vi "array -- bilinear regression 2D -- V1.vi"(7 "action":T2, 10 "fit  IN":dbl[](array[numeric])=[1.9, 2.6, 3.3, 1.0, 2.7, 3.9], 11 "xyz IN":cluster{"x":dbl[], "y":dbl[], "z":dbl[]}={"x"=[0.0, 0.0, 0.0, -1.0, -1.0, -1.0, 1.0, 1.0, 1.0], "y"=[-1.0, 0.0, 1.0, -1.0, 0.0, 1.0, -1.0, 0.0, 1.0], "z"=[1.0, 0.0, 1.0, 4.0, 1.0, 0.0, 0.0, 1.0, 4.0]}) -> (1 "fit map out":map{T1, dbl}(c390)={enum."1"=0.0, enum."x"=0.0, enum."y"=0.0, enum."xx"=1.0, enum."xy"=1.0, enum."yy"=1.0}, 2 "fit OUT":dbl[](array[numeric])=[1.0, 1.0, 1.0, 0.0, 0.0, 0.0], 3 "xyz OUT":cluster{"x":dbl[], "y":dbl[], "z":dbl[]}={"x"=[0.0, 0.0, 0.0, -1.0, -1.0, -1.0, 1.0, 1.0, 1.0], "y"=[-1.0, 0.0, 1.0, -1.0, 0.0, 1.0, -1.0, 0.0, 1.0], "z"=[1.0, 0.0, 1.0, 4.0, 1.0, 0.0, 0.0, 1.0, 4.0]})   [LabVIEW 2021]
uses:
  array -- fit control .ctl
  array -- bilinear regression 2D.ctl
  <vilib>/Analysis/baseanly.llb/Matrix Type of Inverse Matrix.ctl
  <vilib>/Analysis/baseanly.llb/Real A x B.vi
  <vilib>/Analysis/Matrix/Numeric/Conversions/Array To Matrix - RA2.vi
  <vilib>/Analysis/baseanly.llb/Real Inverse Matrix.vi
  <vilib>/Analysis/Matrix/Numeric/Conversions/Matrix To Array - RM.vi
  <vilib>/Analysis/NI_AALBase.lvlib
  <vilib>/Analysis/Matrix/NI_Matrix.lvlib
panel:
  out "y OUT":dbl[](array[numeric])=[-1.0, 0.0, 1.0, -1.0, 0.0, 1.0, -1.0, 0.0, 1.0]
  out "y":dbl[](array[numeric])=[-1.0, 0.0, 1.0, -1.0, 0.0, 1.0, -1.0, 0.0, 1.0]
  out "x OUT":dbl[](array[numeric])=[0.0, 0.0, 0.0, -1.0, -1.0, -1.0, 1.0, 1.0, 1.0]
  out "z OUT":dbl[](array[numeric])=[1.0, 0.0, 1.0, 4.0, 1.0, 0.0, 0.0, 1.0, 4.0]
  out "z":dbl[](array[numeric])=[1.0, 0.0, 1.0, 4.0, 1.0, 0.0, 0.0, 1.0, 4.0]
  out "x":dbl[](array[numeric])=[0.0, 0.0, 0.0, -1.0, -1.0, -1.0, 1.0, 1.0, 1.0]
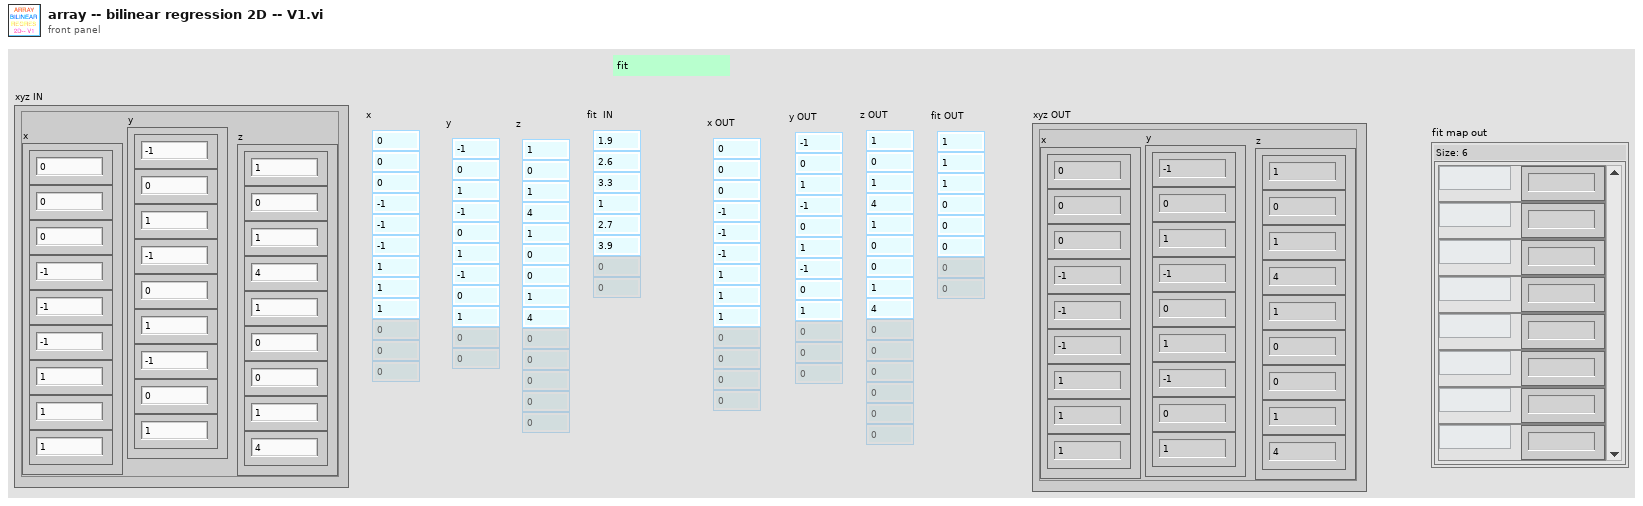
[diagram p1: front panel]
types:
  T1 = typedef "array -- bilinear regression 2D.ctl" = enum16{"1", "x", "y", "xx", "xy", "yy", "xxy", "xyy", "yyy", "xxx", "xxyy", "xyyy", "xxxy", "yyyy", "xxxx", "xxz", "xyz", "yyz", "xz", "yz", "z"}
  T2 = typedef "array -- fit control .ctl" = enum16{"fit", "calc", "check", "init"}
  T3 = typedef "NI_AALBase.lvlib/Matrix Type of Inverse Matrix.ctl" = enum32{"General", "Positive Definite", "Lower Triangular", "Upper Triangular"}
  T4 = typedef "NI_Matrix.lvlib/RealMatrix.ctl" = dbl[][]
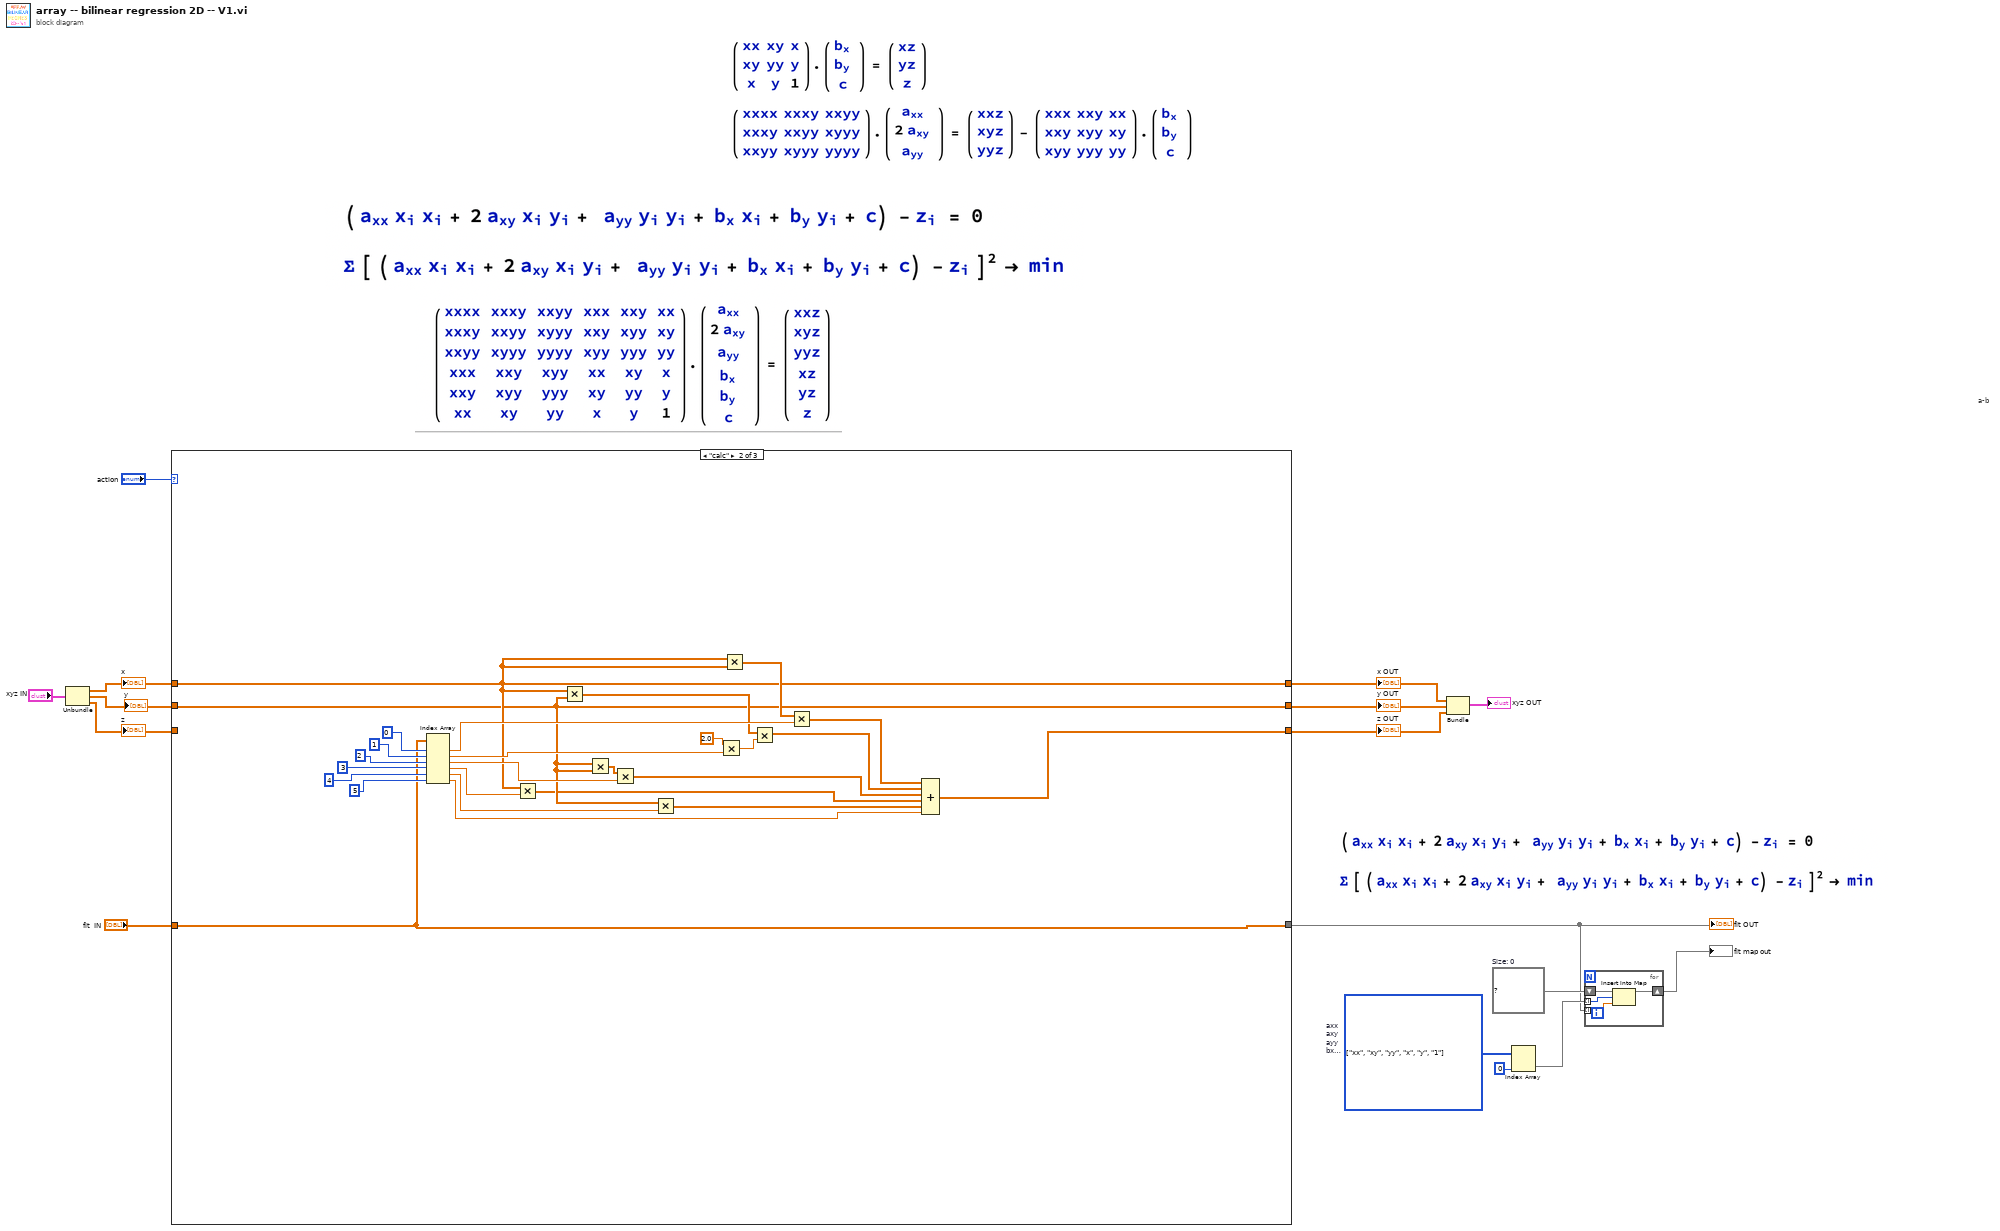
[diagram p0: block diagram]
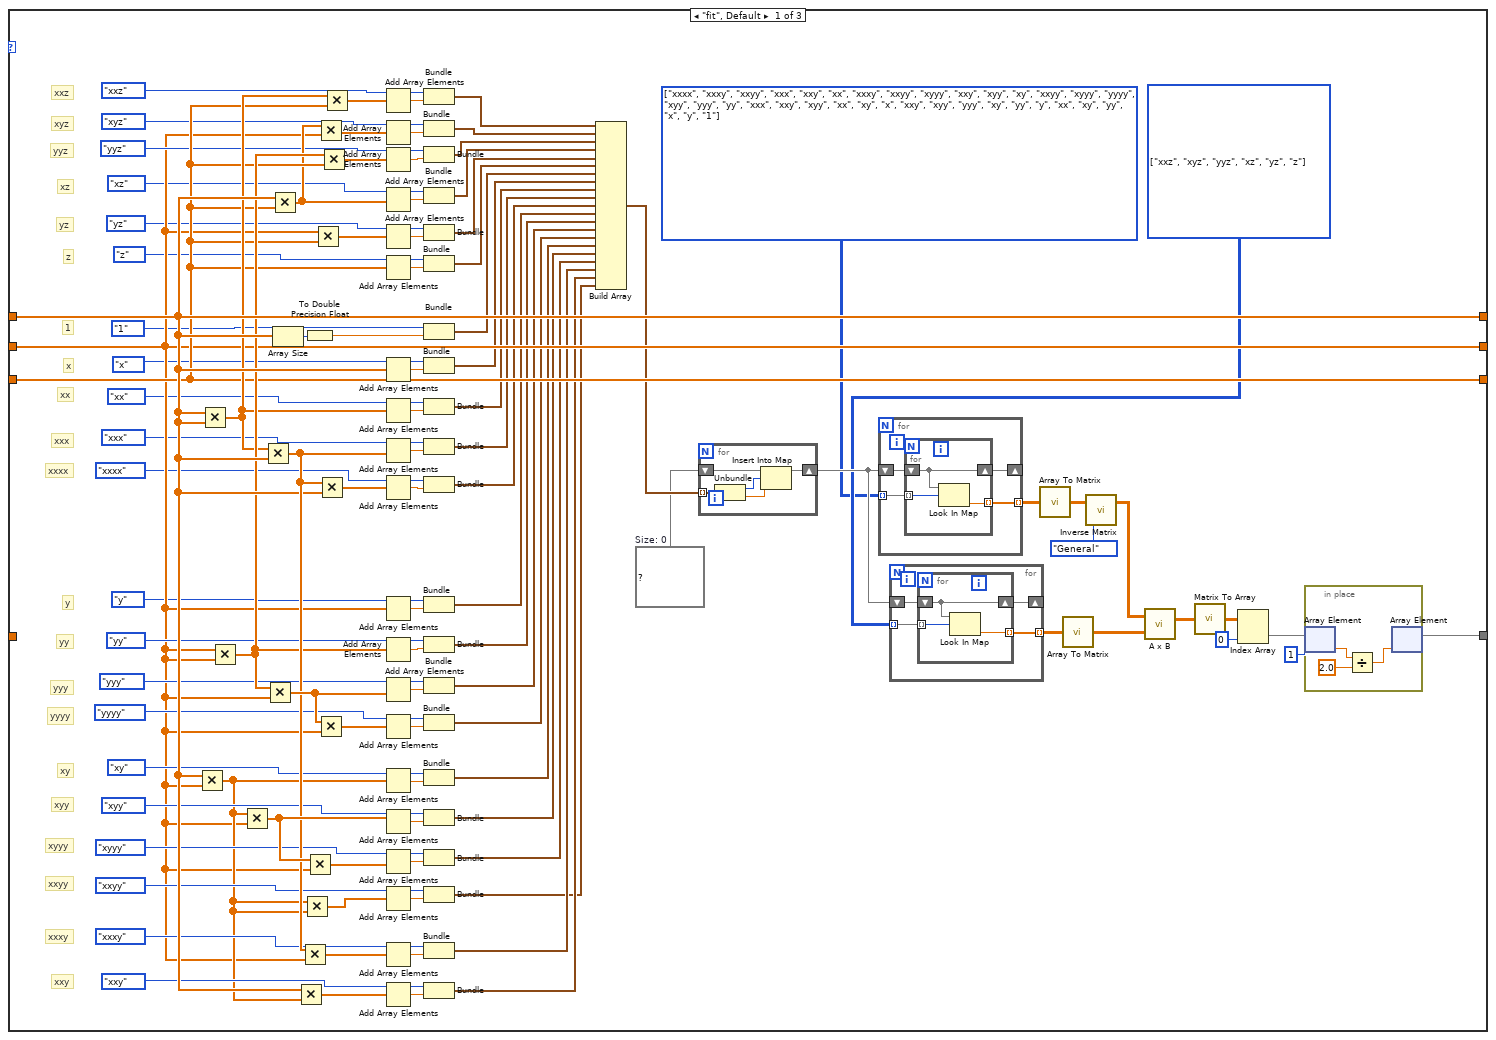
[diagram p2: hidden frame]
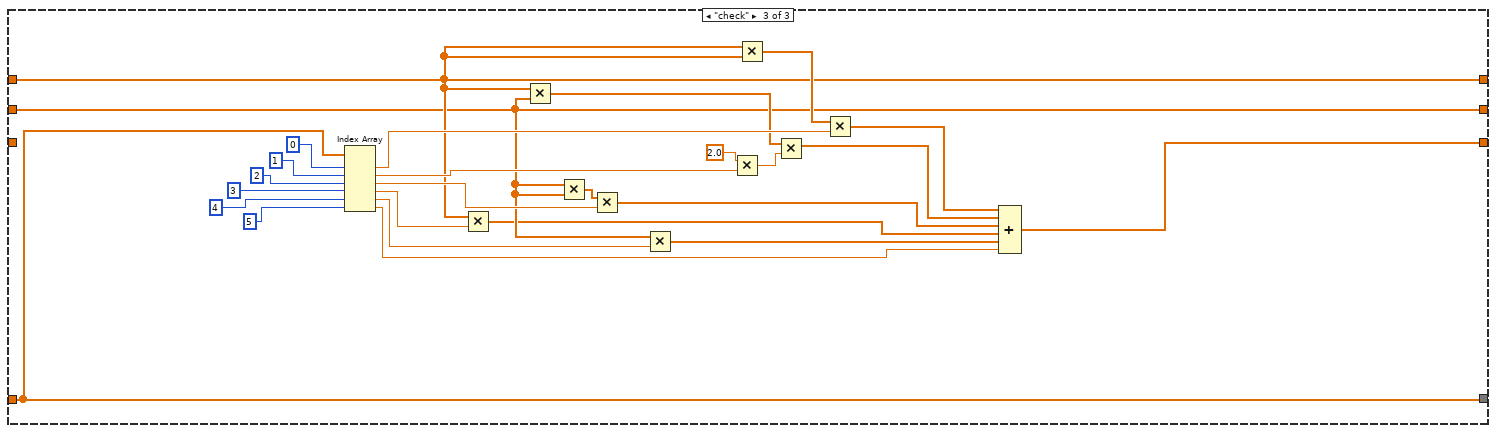
[diagram p3: hidden frame]
diagram:
  w3 = map{T1, dbl} {}  # Size: 0
  w5 = T1[][] [[enum."xx"], [enum."xy"], [enum."yy"], [enum."x"], [enum."y"], [enum."1"]] items=["1", "x", "y", "xx", "xy", "yy", "xxy", "xyy", "yyy", "xxx", "xxyy", "xyyy", "xxxy", "yyyy", "xxxx", "xxz", "xyz", "yyz", "xz", "yz", "z"]  # axx axy ayy bx by c
  # "a-b"
  n1 = Unbundle("xyz IN") -> ("x"=w10:dbl[], "y"=w9:dbl[], "z"=w8:dbl[])
  "x" <- w10
  "z" <- w8
  "y" <- w9
  n2 = case shown="\"calc\"" "action" {
    tunnel: w8 -> [w99 _ _]
    tunnel: w10 -> [w102 w151 w177]
    tunnel: [w20 w140 w166] -> w2
    tunnel: [w99 w141 w167] -> w12
    tunnel: [w102 w151 w177] -> w14
    tunnel: "fit  IN" -> [_ w140 w166]
    tunnel: w9 -> [w71 w148 w174]
    tunnel: [w71 w148 w174] -> w13
    frame "fit", Default {
      w18 = T1[][] [[enum."xxz"], [enum."xyz"], [enum."yyz"], [enum."xz"], [enum."yz"], [enum."z"]] items=["1", "x", "y", "xx", "xy", "yy", "xxy", "xyy", "yyy", "xxx", "xxyy", "xyyy", "xxxy", "yyyy", "xxxx", "xxz", "xyz", "yyz", "xz", "yz", "z"]
      w17 = T1[][] [[enum."xxxx", enum."xxxy", enum."xxyy", enum."xxx", enum."xxy", enum."xx"], [enum."xxxy", enum."xxyy", enum."xyyy", enum."xxy", enum."xyy", enum."xy"], [enum."xxyy", enum."xyyy", enum."yyyy", enum."xyy", enum."yyy", enum."yy"], [enum."xxx", enum."xxy", enum."xyy", enum."xx", enum."xy", enum."x"], [enum."xxy", enum."xyy", enum."yyy", enum."xy", enum."yy", enum."y"], [enum."xx", enum."xy", enum."yy", enum."x", enum."y", enum."1"]] items=["1", "x", "y", "xx", "xy", "yy", "xxy", "xyy", "yyy", "xxx", "xxyy", "xyyy", "xxxy", "yyyy", "xxxx", "xxz", "xyz", "yyz", "xz", "yz", "z"]
      w21 = map{T1, dbl} {}  # Size: 0
      # "z"
      # "xxz"
      # "yz"
      # "xz"
      # "yyz"
      # "xyz"
      # "xxy"
      # "xxxy"
      # "xxyy"
      # "xyyy"
      # "xyy"
      # "xy"
      # "yyyy"
      # "yyy"
      # "yy"
      # "y"
      # "1"
      # "xxxx"
      # "xxx"
      # "xx"
      # "x"
      n3 = Multiply(x=w102, y=w71) -> (x*y=w79:dbl[])
      n4 = Multiply(x=w102, y=w102) -> (x*y=w100:dbl[])
      n5 = Multiply(x=w71, y=w71) -> (x*y=w101:dbl[])
      n6 = Multiply(x=w79, y=w71) -> (x*y=w108:dbl[])
      n7 = Multiply(x=w100, y=w102) -> (x*y=w105:dbl[])
      n8 = Multiply(x=w101, y=w71) -> (x*y=w112:dbl[])
      n9 = Multiply(x=w102, y=w99) -> (x*y=w97:dbl[])
      n10 = Array Size(array=w102) -> (size(s)=w60:i32)
      n11 = Multiply(x=w102, y=w79) -> (x*y=w106:dbl[])
      n12 = Multiply(x=w105, y=w71) -> (x*y=w107:dbl[])
      n13 = Multiply(x=w79, y=w79) -> (x*y=w109:dbl[])
      n14 = To Double Precision Float(number=w60) -> (double precision float=w45:dbl)
      n15 = Multiply(x=w108, y=w71) -> (x*y=w110:dbl[])
      n16 = Multiply(x=w71, y=w99) -> (x*y=w104:dbl[])
      n17 = Multiply(x=w97, y=w71) -> (x*y=w96:dbl[])
      n18 = Multiply(x=w112, y=w71) -> (x*y=w111:dbl[])
      n19 = Multiply(x=w105, y=w102) -> (x*y=w117:dbl[])
      n20 = Multiply(x=w101, y=w99) -> (x*y=w103:dbl[])
      n21 = Multiply(x=w100, y=w99) -> (x*y=w98:dbl[])
      n22 = Add Array Elements(numeric array=w98) -> (sum=w95:dbl)
      n23 = Add Array Elements(numeric array=w96) -> (sum=w93:dbl)
      n24 = Add Array Elements(numeric array=w103) -> (sum=w90:dbl)
      n25 = Add Array Elements(numeric array=w97) -> (sum=w57:dbl)
      n26 = Add Array Elements(numeric array=w104) -> (sum=w55:dbl)
      n27 = Add Array Elements(numeric array=w99) -> (sum=w53:dbl)
      n28 = Add Array Elements(numeric array=w102) -> (sum=w62:dbl)
      n29 = Add Array Elements(numeric array=w100) -> (sum=w63:dbl)
      n30 = Add Array Elements(numeric array=w105) -> (sum=w66:dbl)
      n31 = Add Array Elements(numeric array=w117) -> (sum=w67:dbl)
      n32 = Add Array Elements(numeric array=w71) -> (sum=w70:dbl)
      n33 = Add Array Elements(numeric array=w101) -> (sum=w72:dbl)
      n34 = Add Array Elements(numeric array=w112) -> (sum=w75:dbl)
      n35 = Add Array Elements(numeric array=w111) -> (sum=w77:dbl)
      n36 = Add Array Elements(numeric array=w79) -> (sum=w36:dbl)
      n37 = Add Array Elements(numeric array=w108) -> (sum=w81:dbl)
      n38 = Add Array Elements(numeric array=w110) -> (sum=w83:dbl)
      n39 = Add Array Elements(numeric array=w109) -> (sum=w85:dbl)
      n40 = Add Array Elements(numeric array=w107) -> (sum=w87:dbl)
      n41 = Add Array Elements(numeric array=w106) -> (sum=w88:dbl)
      n42 = Bundle(array_--_bilinear_regression_2D."xxz", "Numeric"=w95) -> (w52:cluster{T1, "Numeric":dbl})  [unwired: 1 in]
      n43 = Bundle(array_--_bilinear_regression_2D."xyz", "Numeric"=w93) -> (w51:cluster{T1, "Numeric":dbl})  [unwired: 1 in]
      n44 = Bundle(array_--_bilinear_regression_2D."yyz", "Numeric"=w90) -> (w50:cluster{T1, "Numeric":dbl})  [unwired: 1 in]
      n45 = Bundle(array_--_bilinear_regression_2D."xz", "Numeric"=w57) -> (w49:cluster{T1, "Numeric":dbl})  [unwired: 1 in]
      n46 = Bundle(array_--_bilinear_regression_2D."yz", "Numeric"=w55) -> (w48:cluster{T1, "Numeric":dbl})  [unwired: 1 in]
      n47 = Bundle(array_--_bilinear_regression_2D."z", "Numeric"=w53) -> (w47:cluster{T1, "Numeric":dbl})  [unwired: 1 in]
      n48 = Bundle(array_--_bilinear_regression_2D."1", w45) -> (w46:cluster{T1, dbl})  [unwired: 1 in]
      n49 = Bundle(array_--_bilinear_regression_2D."x", "Numeric"=w62) -> (w44:cluster{T1, "Numeric":dbl})  [unwired: 1 in]
      n50 = Bundle(array_--_bilinear_regression_2D."xx", "Numeric"=w63) -> (w43:cluster{T1, "Numeric":dbl})  [unwired: 1 in]
      n51 = Bundle(array_--_bilinear_regression_2D."xxx", "Numeric"=w66) -> (w42:cluster{T1, "Numeric":dbl})  [unwired: 1 in]
      n52 = Bundle(array_--_bilinear_regression_2D."xxxx", "Numeric"=w67) -> (w41:cluster{T1, "Numeric":dbl})  [unwired: 1 in]
      n53 = Bundle(array_--_bilinear_regression_2D."y", "Numeric"=w70) -> (w40:cluster{T1, "Numeric":dbl})  [unwired: 1 in]
      n54 = Bundle(array_--_bilinear_regression_2D."yy", "Numeric"=w72) -> (w22:cluster{T1, "Numeric":dbl})  [unwired: 1 in]
      n55 = Bundle(array_--_bilinear_regression_2D."yyy", "Numeric"=w75) -> (w39:cluster{T1, "Numeric":dbl})  [unwired: 1 in]
      n56 = Bundle(array_--_bilinear_regression_2D."yyyy", "Numeric"=w77) -> (w38:cluster{T1, "Numeric":dbl})  [unwired: 1 in]
      n57 = Bundle(array_--_bilinear_regression_2D."xy", "Numeric"=w36) -> (w37:cluster{T1, "Numeric":dbl})  [unwired: 1 in]
      n58 = Bundle(array_--_bilinear_regression_2D."xyy", "Numeric"=w81) -> (w35:cluster{T1, "Numeric":dbl})  [unwired: 1 in]
      n59 = Bundle(array_--_bilinear_regression_2D."xyyy", "Numeric"=w83) -> (w34:cluster{T1, "Numeric":dbl})  [unwired: 1 in]
      n60 = Bundle(array_--_bilinear_regression_2D."xxyy", "Numeric"=w85) -> (w31:cluster{T1, "Numeric":dbl})  [unwired: 1 in]
      n61 = Bundle(array_--_bilinear_regression_2D."xxxy", "Numeric"=w87) -> (w33:cluster{T1, "Numeric":dbl})  [unwired: 1 in]
      n62 = Bundle(array_--_bilinear_regression_2D."xxy", "Numeric"=w88) -> (w32:cluster{T1, "Numeric":dbl})  [unwired: 1 in]
      n63 = Build Array(w52, w51, w50, w49, w48, w47, w46, w44, w43, w42, w41, w40, w22, w39, w38, w37, w35, w34, w33, w32, w31) -> (w30:cluster{T1, "Numeric":dbl}[])
      n64 = for {
        tunnel: w30 -> [w130] mode=indexing
        shift-right: [w131] -> w19
        shift-left: w21 -> [w132]
        n65 = Unbundle(w130) -> (w129:T1, "Numeric"=w128:dbl)
        n66 = Insert Into Map(map in=w132, key=w129, value=w128) -> (map out=w131:map{T1, dbl})  [unwired: 2 out]
      }
      n67 = for {
        tunnel: w17 -> [w136] mode=indexing
        shift-right: [w134] -> _
        shift-left: w19 -> [w135]
        tunnel: [w133] -> w28 mode=indexing
        n68 = for {
          tunnel: w136 -> [w138] mode=indexing
          shift-right: [w139] -> w134
          shift-left: w135 -> [w139]
          tunnel: [w137] -> w133 mode=indexing
          n69 = Look In Map(map=w139, key=w138) -> (value=w137:dbl)  [unwired: 1 in, 1 out]
        }
      }
      n70 = for {
        shift-right: [w123] -> _
        shift-left: w19 -> [w124]
        tunnel: w18 -> [w122] mode=indexing
        tunnel: [w121] -> w27 mode=indexing
        n71 = for {
          shift-right: [w127] -> w123
          shift-left: w124 -> [w127]
          tunnel: w122 -> [w126] mode=indexing
          tunnel: [w125] -> w121 mode=indexing
          n72 = Look In Map(map=w127, key=w126) -> (value=w125:dbl)  [unwired: 1 in, 1 out]
        }
      }
      n73 = call-poly <vilib>:"Array To Matrix.vi"("Real 2D Array"=w28) -> ("Real Matrix"=w23:T4)
      n74 = call-poly <vilib>:"Array To Matrix.vi"("Real 2D Array"=w27) -> ("Real Matrix"=w26:T4)
      n75 = call-poly <vilib>:"Inverse Matrix.vi"("matrix type"=Matrix_Type_of_Inverse_Matrix."General", "Input Matrix"=w23) -> ("Inverse Matrix"=w116:T4)  [unwired: 1 out]
      n76 = call-poly <vilib>:"A x B.vi"("B"=w26, "A"=w116) -> ("A x B"=w115:T4)  [unwired: 1 out]
      n77 = call-poly <vilib>:"Matrix To Array.vi"("Real Matrix"=w115) -> ("Real 2D Array"=w114:dbl[][])
      n78 = Index Array(array=w114, index (col)=0 ("disabled index (col)")) -> (element=w25:dbl[])  [unwired: 1 in]
      n79 = in-place {
        n80 = in-place-array #1(w25, 1) -> (w120:dbl)
        n81 = Divide(x=w120, y=2.0) -> (x/y=w118:dbl)
        n82 = in-place-array #1(w118) -> (w20:dbl[])  [unwired: 1 out]
      }
    }
    frame "calc" {
      n83 = Index Array(array=w140, index #1=0 ("index"), index #2=1 ("index"), index #3=2 ("index"), index #4=3 ("index"), index #5=4 ("index"), index #6=5 ("index")) -> (element #1=w158:dbl, element #2=w152:dbl, element #3=w154:dbl, element #4=w150:dbl, element #5=w149:dbl, element #6=w142:dbl)
      n84 = Multiply(x=w151, y=w150) -> (x*y=w144:dbl[])
      n85 = Multiply(x=w151, y=w148) -> (x*y=w157:dbl[])
      n86 = Multiply(x=w148, y=w148) -> (x*y=w155:dbl[])
      n87 = Multiply(x=w155, y=w154) -> (x*y=w145:dbl[])
      n88 = Multiply(x=w148, y=w149) -> (x*y=w143:dbl[])
      n89 = Multiply(x=2.0 ("y"), y=w152) -> (x*y=w156:dbl)
      n90 = Multiply(x=w151, y=w151) -> (x*y=w159:dbl[])
      n91 = Multiply(x=w157, y=w156) -> (x*y=w146:dbl[])
      n92 = Multiply(x=w159, y=w158) -> (x*y=w147:dbl[])
      n93 = Compound Arithmetic op=ADD(w147, w146, w145, w144, w143, w142) -> (w141:dbl[])
    }
    frame "check" {
      n94 = Index Array(array=w166, index #1=0 ("index"), index #2=1 ("index"), index #3=2 ("index"), index #4=3 ("index"), index #5=4 ("index"), index #6=5 ("index")) -> (element #1=w184:dbl, element #2=w178:dbl, element #3=w180:dbl, element #4=w176:dbl, element #5=w175:dbl, element #6=w168:dbl)
      n95 = Multiply(x=w177, y=w176) -> (x*y=w170:dbl[])
      n96 = Multiply(x=w177, y=w174) -> (x*y=w183:dbl[])
      n97 = Multiply(x=w174, y=w174) -> (x*y=w181:dbl[])
      n98 = Multiply(x=w181, y=w180) -> (x*y=w171:dbl[])
      n99 = Multiply(x=w174, y=w175) -> (x*y=w169:dbl[])
      n100 = Multiply(x=2.0 ("y"), y=w178) -> (x*y=w182:dbl)
      n101 = Multiply(x=w177, y=w177) -> (x*y=w185:dbl[])
      n102 = Multiply(x=w183, y=w182) -> (x*y=w172:dbl[])
      n103 = Multiply(x=w185, y=w184) -> (x*y=w173:dbl[])
      n104 = Compound Arithmetic op=ADD(w173, w172, w171, w170, w169, w168) -> (w167:dbl[])
    }
  }
  "fit OUT" <- w2
  "z OUT" <- w12
  "x OUT" <- w14
  "y OUT" <- w13
  n105 = Bundle("x"=w14, "y"=w13, "z"=w12) -> (→"xyz OUT":cluster{"x":dbl[], "y":dbl[], "z":dbl[]})  [unwired: 1 in]
  n106 = Index Array(array=w5, index (col)=0 ("disabled index (col)")) -> (element=w6:T1[])  [unwired: 1 in]
  n107 = for {
    shift-right: [w194] -> w1
    shift-left: w3 -> [w195]
    tunnel: w6 -> [w193] mode=indexing
    tunnel: w2 -> [w192] mode=indexing
    n108 = Insert Into Map(map in=w195, key=w193, value=w192) -> (map out=w194:map{T1, dbl})  [unwired: 2 out]
  }
  "fit map out" <- w1
